vi "Default Settings.vi"(8 "error in (no error)":errorcluster, 11 "8 Inch CAD Dispense in":refnum<class "8 Inch CAD Dispense.lvclass">) -> (0 "error out":errorcluster, 3 "8 Inch CAD Dispense out":refnum<class "8 Inch CAD Dispense.lvclass">)   [LabVIEW 2020, in "8 Inch CAD Dispense.lvclass"]
uses:
  8 Inch CAD Dispense.lvclass
  C:/Users/HEP/Documents/Aerotech gantry/UCSB-Gantry-master-main/V5/Classes/Routine/Dispense/CAD Dispense/CAD Dispense.lvclass
  C:/Users/HEP/Documents/Aerotech gantry/UCSB-Gantry-master-main/V5/Classes/Routine/Dispense/Dispense.lvclass
  CAD Dispense.lvclass/CAD Dispense.ctl
  Read Glue Speed.vi
  Read Move Speed.vi
  CAD Dispense.lvclass
  Dispense.lvclass
panel:
  # "This Routine does not Accept Settings"
  # "This Routine Does not Accept Settings"
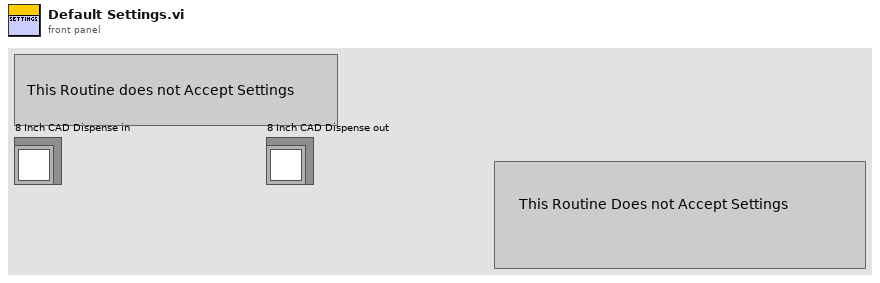
[diagram p1: front panel]
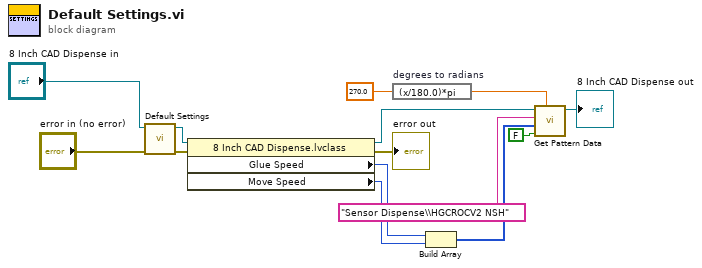
[diagram p0: block diagram]
diagram:
  n1 = call-parent "Default Settings.vi"("error in (no error)"="error in (no error)", "CAD Dispense in"="8 Inch CAD Dispense in") -> ("error out"=w2:errorcluster, "CAD Dispense out"=w12:refnum<class "8 Inch CAD Dispense.lvclass">)  [unwired: 8 in]
  n2 = property class="8 Inch CAD Dispense.lvclass"(reference=w12, error in=w2) -> (reference out=w8:refnum<class "8 Inch CAD Dispense.lvclass">, error out=→"error out":errorcluster, "Glue Speed"=w11:i32, "Move Speed"=w10:i32)
  n3 = expression code="(x/180.0)*pi" "degrees to radians"(270.0) -> (w5:dbl)
  n4 = Build Array(w11, w10) -> (w9:i32[])
  n5 = call "Get Pattern Data.vi"("theta"=w5, "Iterative?"=FALSE, "File Name"=w9, "Folder Name"="Sensor Dispense\\HGCROCV2 NSH", "Dispense.lvclass"=w8) -> ("Dispense Out"=→"8 Inch CAD Dispense out":refnum<class "8 Inch CAD Dispense.lvclass">)  [unwired: 6 in]
